vi "ISEG_HVChannel.ProcEvents.vi"(0 "i ref in":refnum<vi>, 5 "error in (no error)":errorcluster) -> (14 "i ref out":refnum<vi>, 19 "error out":errorcluster)   [LabVIEW 2014, in "ISEG_HVChannel.lvlib"]
doc: "This method is used to define the events the object will listen to. Add your own events here."
uses:
  ISEG_HVChannel.lvlib
  CSCore/BaseProcess/BaseProcess.event definition.ctl
  CSCore/CAEObj/CAEObj.event definition.ctl
  CSCore/BaseProcess/BaseProcess.descriptor string definition.ctl
  CSCore/BaseProcess/BaseProcess.lvlib
  CSCore/CAEObj/CAEObj.lvlib
panel:
  in  "event definition":T1={"CAEEvtDef"={"URL"="lvmsg://setKill", "enable"=TRUE, "ignoreResID"=FALSE}, "Data Descriptor"="S:1 n[Kill] //If Kill=True: Switch OFF at the max rate all system channels;"}
  in  "event definition":T1={"CAEEvtDef"={"URL"="lvmsg://setKill", "enable"=TRUE, "ignoreResID"=FALSE}, "Data Descriptor"="S:1 n[Kill] //If Kill=True: Switch OFF at the max rate all system channels;"}
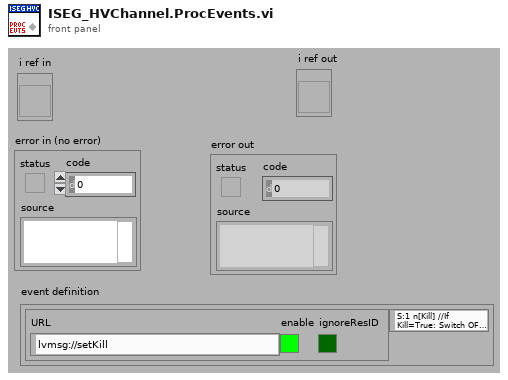
[diagram p1: front panel]
types:
  T1 = typedef "BaseProcess.lvlib/BaseProcess.event definition.ctl" = cluster{"CAEEvtDef":T2, "Data Descriptor":T3}
  T2 = typedef "CAEObj.lvlib/CAEObj.event definition.ctl" = cluster{"URL":string, "enable":bool, "ignoreResID":bool}
  T3 = typedef "BaseProcess.lvlib/BaseProcess.descriptor string definition.ctl" = string
  T4 = typedef "ISEG_HVChannel.lvlib/ISEG_HVChannel.i attribute.ctl" = cluster{"Channel Array":cluster{"Logical Name":string, "Address":string, "error in (no error)":errorcluster, "Status":cluster{"Status":i16, "DIM Status":T5}, "On":cluster{"On":bool, "DIM Status":T5}, "VMeas ":cluster{"VMeas":dbl, "DIM Status":T5}, "VSet ":cluster{"VSet":dbl, "DIM Status":T5}, "ITrip ":cluster{"ITrip":dbl, "DIM Status":T5}, "IMeas":cluster{"IMeas":dbl, "DIM Status":T5}, " RampSpeed":cluster{"RampSpeed":dbl, "DIM Status":T5}, "EventMask ":cluster{"EventMask":i16, "DIM Status":T5}}[], "VoltageInRangeBand":dbl, "NofCh":cluster{"NofCh":i32, "DIM Service":i32}, "BoardPrefix":string}
  T5 = typedef "ISEG_HVChannel.lvlib/ISEG_HVChannel.DIM Status.ctl" = cluster{"no link":bool, "quality":i32, "Time Stamp":timestamp}
  T6 = cluster{"Logical Name":string, "Address":string, "error in (no error)":errorcluster, "Status":cluster{"Status":i16, "DIM Status":T5}, "On":cluster{"On":bool, "DIM Status":T5}, "VMeas ":cluster{"VMeas":dbl, "DIM Status":T5}, "VSet ":cluster{"VSet":dbl, "DIM Status":T5}, "ITrip ":cluster{"ITrip":dbl, "DIM Status":T5}, "IMeas":cluster{"IMeas":dbl, "DIM Status":T5}, " RampSpeed":cluster{"RampSpeed":dbl, "DIM Status":T5}, "EventMask ":cluster{"EventMask":i16, "DIM Status":T5}}[]
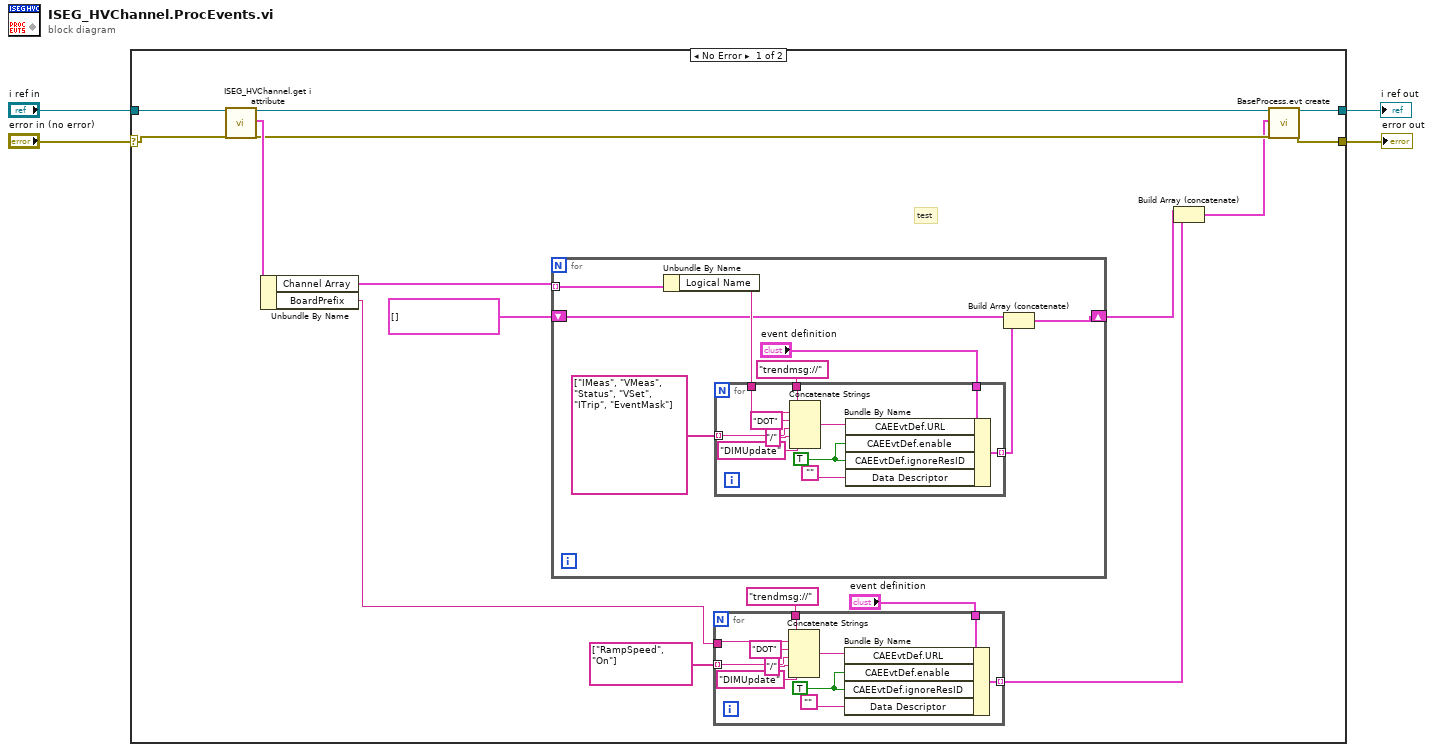
[diagram p0: block diagram]
diagram:
  n1 = case shown="No Error" "error in (no error)" {
    selector: "error in (no error)" -> [w5 w51]
    tunnel: "i ref in" -> [w18 w52]
    tunnel: [w20 w52] -> w3
    tunnel: [w19 w51] -> w2
    frame No Error {
      # "test"
      n2 = call "ISEG_HVChannel.get i attribute.vi"("i ref in"=w18, "error in (no error)"=w5) -> ("i ref out"=w16:refnum<vi>, "i attribute"=w17:T4, "error out"=w15:errorcluster)  [unwired: 15 in]
      n3 = Unbundle By Name(w17) -> ("Channel Array"=w11:T6, "BoardPrefix"=w6:string)
      n4 = for {
        tunnel: w11 -> [w36] mode=indexing
        shift-right: [w33] -> w13
        shift-left: T1[] [] -> [w35]
        n5 = Unbundle By Name(w36) -> ("Logical Name"=w37:string)
        n6 = for {
          tunnel: "event definition" -> [w50]
          tunnel: "trendmsg://" -> [w49]
          tunnel: [w44] -> w34 mode=indexing
          tunnel: w37 -> [w42]
          tunnel: string[] ["IMeas", "VMeas", "Status", "VSet", "ITrip", "EventMask"] -> [w40] mode=indexing
          w47 = TRUE ("CAEEvtDef.ignoreResID")
          n7 = Concatenate Strings(w49, w42, "DOT" ("string"), w40, "/" ("string"), "DIMUpdate" ("string")) -> (w48:string)
          n8 = Bundle By Name(cluster=w50, "CAEEvtDef.URL"=w48, "CAEEvtDef.enable"=w47, "CAEEvtDef.ignoreResID"=w47, "Data Descriptor"="") -> (w44:T1)
        }
        n9 = Build Array (concatenate)(w35, w34) -> (w33:T1[])
      }
      n10 = for {
        tunnel: "event definition" -> [w31]
        tunnel: "trendmsg://" -> [w30]
        tunnel: [w25] -> w7 mode=indexing
        tunnel: string[] ["RampSpeed", "On"] -> [w22] mode=indexing
        tunnel: w6 -> [w21]
        w28 = TRUE ("CAEEvtDef.ignoreResID")
        n11 = Concatenate Strings(w30, w21, "DOT" ("string"), w22, "/" ("string"), "DIMUpdate" ("string")) -> (w29:string)
        n12 = Bundle By Name(cluster=w31, "CAEEvtDef.URL"=w29, "CAEEvtDef.enable"=w28, "CAEEvtDef.ignoreResID"=w28, "Data Descriptor"="") -> (w25:T1)
      }
      n13 = Build Array (concatenate)(w13, w7) -> (w12:T1[])
      n14 = call "BaseProcess.evt create.vi"("i ref in"=w16, "newEvents"=w12, "error in (no error)"=w15) -> ("i ref out"=w20:refnum<vi>, "error out"=w19:errorcluster)  [unwired: 13 in, 2 out]
    }
    frame Error {
    }
  }
  "i ref out" <- w3
  "error out" <- w2
